vi "SetSystemDefinitionPropertyValueErrorMessage.vi"(8 "error in (no error)":errorcluster, 10 "successful?":bool, 11 "property name":string) -> (0 "error out":errorcluster)   [LabVIEW 2016, in "VeriStandTestUtilities.lvlib"]
uses:
  VeriStandTestUtilities.lvlib
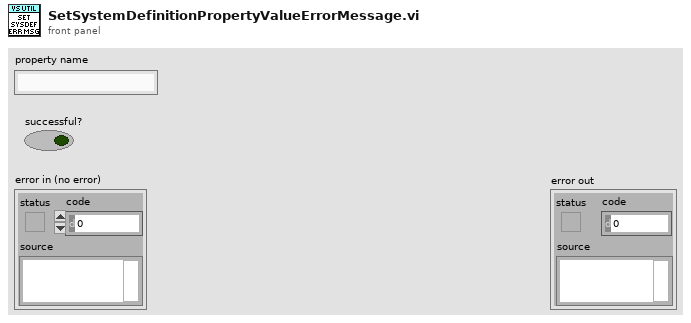
[diagram p1: front panel]
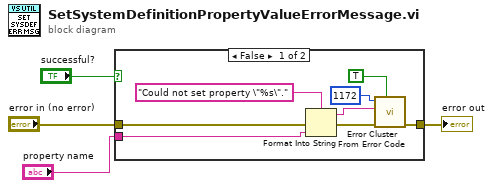
[diagram p0: block diagram]
diagram:
  n1 = case shown="False" "successful?" {
    tunnel: "error in (no error)" -> [w11 w13]
    tunnel: [w10 w13] -> w3
    tunnel: "property name" -> [w6 _]
    frame False {
      n2 = Format Into String(format string="Could not set property \"%s\".", error in=w11, w6) -> (resulting string=w8:string, error out=w9:errorcluster)  [unwired: 1 in]
      n3 = call <vilib>:"Error Cluster From Error Code.vi"("show call chain? (False)"=TRUE, "error in (no error)"=w9, "error message (\"\")"=w8, "error code (0)"=1172) -> ("error out"=w10:errorcluster)  [unwired: 5 in]
    }
    frame True {
    }
  }
  "error out" <- w3
